vi "SSL_CTX_get_cert_store.vi"(8 "error in (no error)":errorcluster, 11 "SSL-Context in":refnum<class "SSL-Context.lvclass">) -> (0 "error out":errorcluster, 2 "X509 Cert Store":u64, 3 "SSL-Context out":refnum<class "SSL-Context.lvclass">)   [LabVIEW 2013, in "SSL_Lib.lvlib" / "SSL-Context.lvclass"]
uses:
  SSL-Context.lvclass
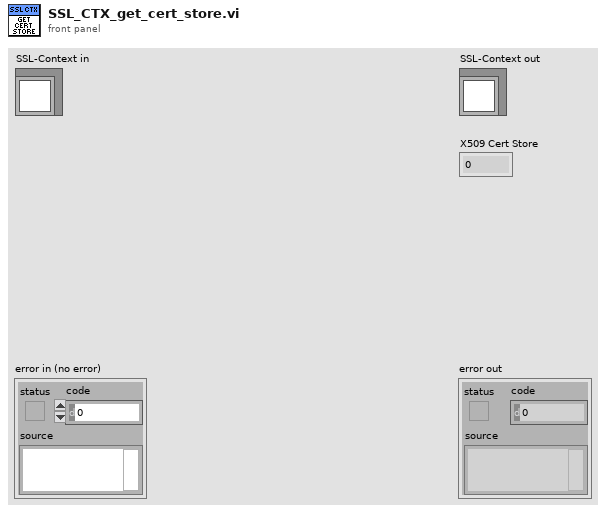
[diagram p1: front panel]
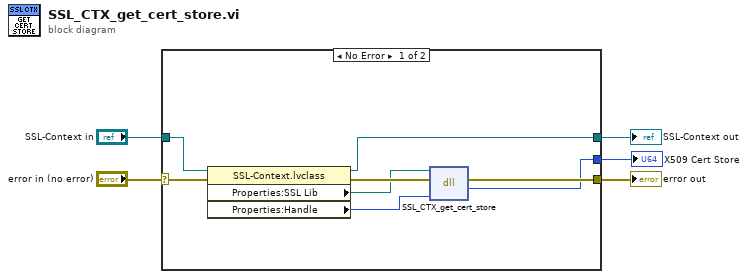
[diagram p0: block diagram]
diagram:
  n1 = case shown="No Error" "error in (no error)" {
    selector: "error in (no error)" -> [w13 w15]
    tunnel: [w8 w15] -> w4
    tunnel: [w7 w14] -> w2
    tunnel: "SSL-Context in" -> [w11 w14]
    tunnel: [w6 _] -> w1
    frame No Error {
      n2 = property class="SSL-Context.lvclass"(reference=w11, error in=w13) -> (reference out=w7:refnum<class "SSL-Context.lvclass">, error out=w12:errorcluster, "Properties:SSL Lib"=w10:path, "Properties:Handle"=w9:u64)
      n3 = dll-call lib="C:/Program Files (x86)/National Instruments/Shared/nissl/NIssleay32.dll" fn="SSL_CTX_get_cert_store"(path in=w10, error in=w12, "SSL_CTX"=w9) -> (error out=w8:errorcluster, "return type"=w6:u64)  [unwired: 2 in, 1 out]
    }
    frame Error {
    }
  }
  "error out" <- w4
  "SSL-Context out" <- w2
  "X509 Cert Store" <- w1
